vi "Close.vi"(8 "error in (no error)":errorcluster, 11 "Query Result in":refnum<class "DapperResult.lvclass">) -> (0 "error out":errorcluster)   [LabVIEW 2020, in "ORM_Dapper.lvlib" / "DapperResult.lvclass"]
uses:
  DapperResult.lvclass
  DapperResult.lvclass/DapperResult.ctl
  Read ref.vi
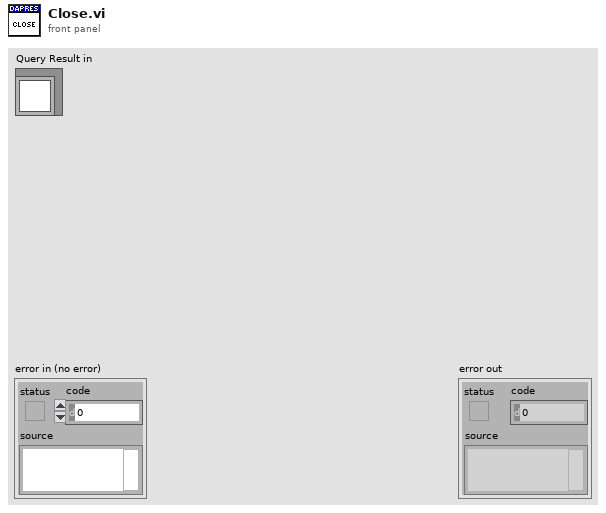
[diagram p1: front panel]
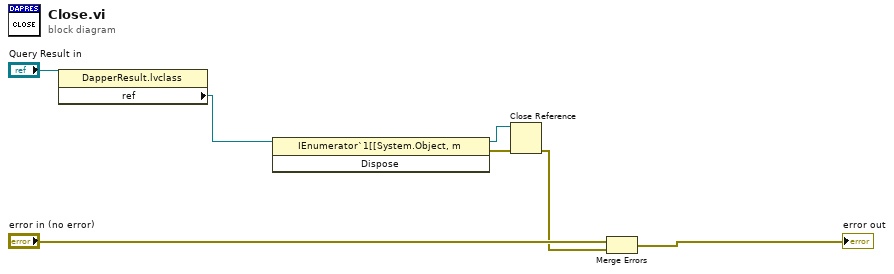
[diagram p0: block diagram]
diagram:
  n1 = property class="DapperResult.lvclass"(reference="Query Result in") -> ("ref"=w1:refnum<k24>)  [unwired: 1 in, 2 out]
  n2 = invoke class="IEnumerator`1[[System.Object, m" method="Dispose"(reference=w1) -> (reference out=w5:refnum<k24>, error out=w6:errorcluster)  [unwired: 2 in, 1 out]
  n3 = Close Reference(reference=w5, error in (no error)=w6) -> (error out=w3:errorcluster)
  n4 = Merge Errors("error in (no error)", w3) -> (→"error out":errorcluster)
